vi "Find Contact.vi"(8 "error in (no error)":errorcluster, 10 "ID":u32, 11 "Data":T1[](array[typedef])) -> (0 "error out":errorcluster, 2 "Index":i32, 3 "dup Data":T1[](array[typedef]))   [LabVIEW 2014, in "Contact Data.lvlib"]
doc: "Searches the data store for a single contact by ID."
uses:
  Contact Data.lvlib
  Contact.ctl
  Position.ctl
  Controls.ctl
  DestinationCluster.ctl
  DesinationControls.ctl
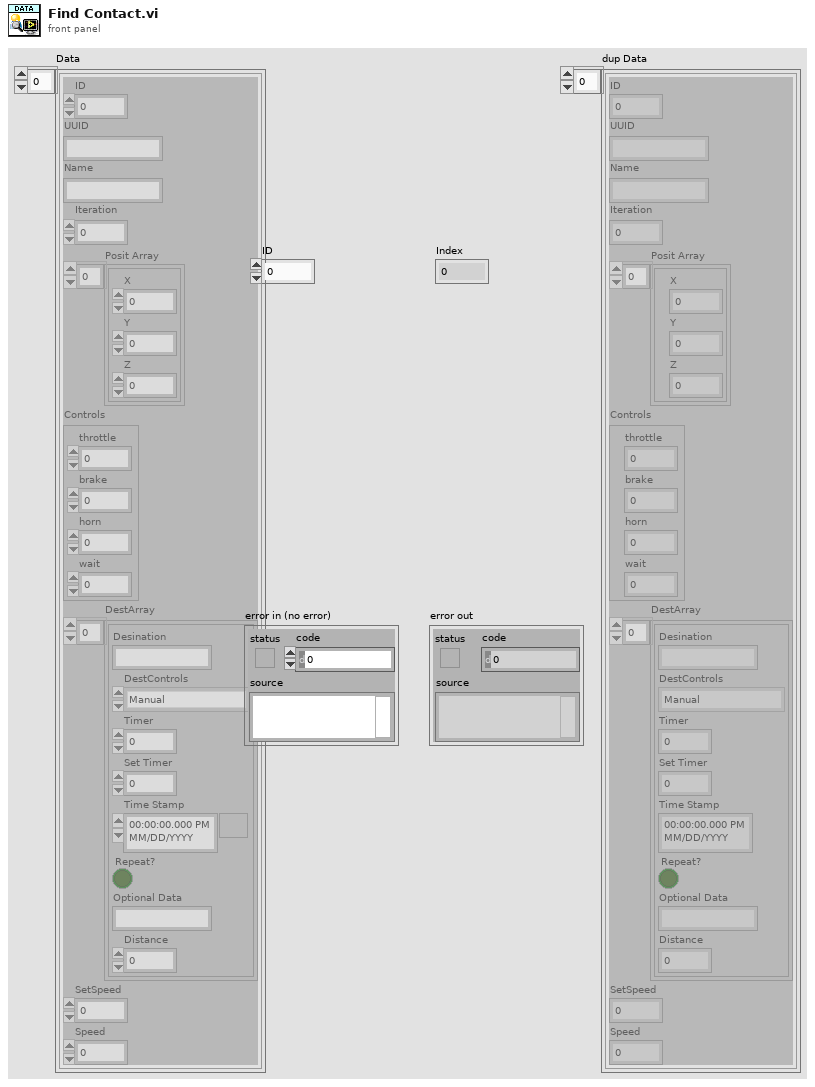
[diagram p1: front panel]
types:
  T1 = typedef "Contact Data.lvlib/Contact.ctl" = cluster{"ID":u32, "UUID":string, "Name":string, "Iteration":i32, "Posit Array":T2[], "Controls":T3, "DestArray":T4[], "SetSpeed":dbl, "Speed":dbl}
  T2 = typedef "Contact Data.lvlib/Position.ctl" = cluster{"X":dbl, "Y":dbl, "Z":dbl}
  T3 = typedef "Contact Data.lvlib/Controls.ctl" = cluster{"throttle":dbl, "brake":dbl, "horn":dbl, "wait":dbl}
  T4 = typedef "Contact Data.lvlib/DestinationCluster.ctl" = cluster{"Desination":string, "DestControls":T5, "Timer":u32, "Set Timer":u32, "Time Stamp":timestamp, "Repeat?":bool, "Optional Data":string, "Distance":dbl}
  T5 = typedef "Contact Data.lvlib/DesinationControls.ctl" = enum16{"Tracker", "Manual", "Stop", "Station DateTime", "Station Timer", "Maintain"}
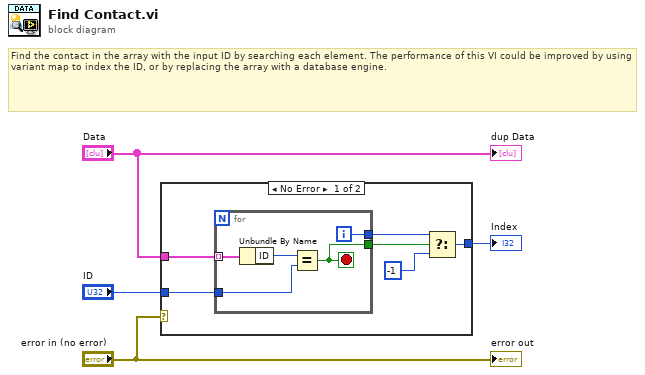
[diagram p0: block diagram]
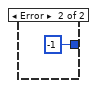
[diagram p2: hidden frame]
diagram:
  # "Find the contact in the array with the input ID by searching each element. The performance of this VI could be improved by using variant map to index the ID, or by replacing the array with a database engine."
  n1 = case shown="No Error" "error in (no error)" {
    tunnel: "ID" -> [w10 _]
    tunnel: "Data" -> [w9 _]
    tunnel: [w5 -1 ("f")] -> w2
    frame No Error {
      n2 = for {
        tunnel: w9 -> [w15] mode=indexing
        tunnel: w10 -> [w13]
        tunnel: [w12] -> w7
        tunnel: [w11] -> w8
        i -> [w12]
        stop <- w11 stop-if-true
        n3 = Unbundle By Name(w15) -> ("ID"=w14:u32)
        n4 = Equal?(x=w14, y=w13) -> (x = y?=w11:bool)
      }
      n5 = Select(t=w7, s=w8, f=-1) -> (s? t:f=w5:i32)
    }
    frame Error {
    }
  }
  "Index" <- w2
  "error out" <- "error in (no error)"
  "dup Data" <- "Data"
